vi "Server_OpenServer.vi"(8 "error in (no error)":errorcluster, 9 "Wait for connection?":bool, 11 "Server":path) -> (0 "error out":errorcluster)   [LabVIEW 2020]
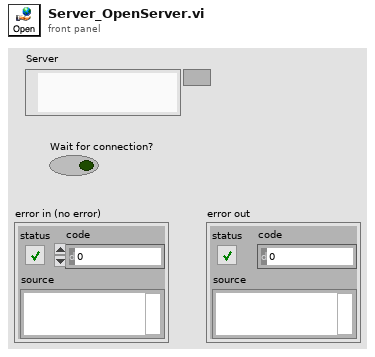
[diagram p1: front panel]
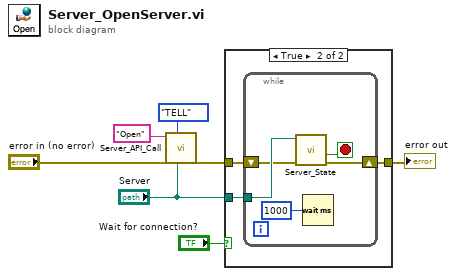
[diagram p0: block diagram]
diagram:
  n1 = call "Server_API_Call.vi"("Server"="Server", "Direction"=enum16{"ASK", "TELL"}."TELL", "error in (no error)"="error in (no error)", "cmd"="Open" ("url")) -> ("error out"=w3:errorcluster)  [unwired: 5 in, 2 out]
  n2 = case shown="True" "Wait for connection?" {
    tunnel: "Server" -> [_ w11]
    tunnel: w3 -> [w8 w10]
    tunnel: [w8 w9] -> w2
    frame False {
    }
    frame True {
      n3 = while {
        tunnel: w11 -> [w16]
        shift-right: [w14] -> w9
        shift-left: w10 -> [w15]
        stop <- w12 stop-if-true
        n4 = call "Server_State.vi"("error in (no error)"=w15, "Server"=w16) -> ("error out"=w14:errorcluster, "Connected?"=w12:bool)  [unwired: 7 in, 1 out]
        n5 = Wait (ms)(milliseconds to wait=u32 1000) -> ()  [unwired: 1 out]
      }
    }
  }
  "error out" <- w2
